vi "Create.vi"(10 "Task ID":string) -> (3 "DataHandlerIdentity out":refnum<class "DataHandlerIdentity.lvclass">)   [LabVIEW 2020, in "VolatusData.lvlib" / "DataHandlerIdentity.lvclass"]
uses:
  DataHandlerIdentity.lvclass
  DataHandlerIdentity.lvclass/DataHandlerIdentity.ctl
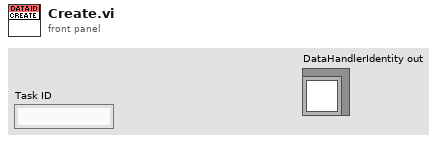
[diagram p1: front panel]
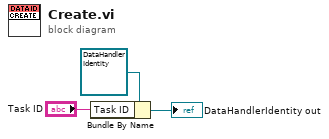
[diagram p0: block diagram]
diagram:
  n1 = Bundle By Name(cluster=refnum<class "DataHandlerIdentity.lvclass"> refnum ("DataHandlerIdentity in"), "Task ID"="Task ID") -> (→"DataHandlerIdentity out":refnum<class "DataHandlerIdentity.lvclass">)
